vi "Boolean Array to Hex Values.vi"(11 "Array in":bool[][](array[boolean])) -> (3 "Array out":u8[](array[numeric]))   [LabVIEW 2026, in "LED Matrix.lvlib" / "Content.lvclass"]
uses:
  Content.lvclass
  Content.lvclass/Content.ctl
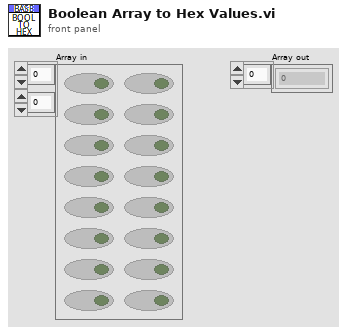
[diagram p1: front panel]
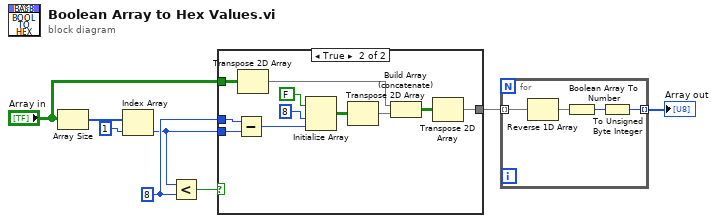
[diagram p0: block diagram]
diagram:
  w4 = 8 ("y")
  n1 = Array Size(array="Array in") -> (size(s)=w7:i32[])
  n2 = Index Array(array=w7, index=1) -> (element=w3:i32)
  n3 = Less?(x=w3, y=w4) -> (x < y?=w5:bool)
  n4 = case shown="True" w5 {
    tunnel: w4 -> [_ w20]
    tunnel: w3 -> [_ w19]
    tunnel: "Array in" -> [w9 w15]
    tunnel: [w9 w10] -> w1
    frame False {
    }
    frame True {
      n5 = Subtract(x=w20, y=w19) -> (x-y=w17:i32)
      n6 = Transpose 2D Array(2D array=w15) -> (transposed array=w12:bool[][])
      n7 = Initialize Array(FALSE, 8 ("dimension size"), w17) -> (w14:bool[][])
      n8 = Transpose 2D Array(2D array=w14) -> (transposed array=w13:bool[][])
      n9 = Build Array (concatenate)(w12, w13) -> (w11:bool[][])
      n10 = Transpose 2D Array(2D array=w11) -> (transposed array=w10:bool[][])
    }
  }
  n11 = for {
    tunnel: [w23] -> w8 mode=indexing
    tunnel: w1 -> [w21] mode=indexing
    n12 = Reverse 1D Array(array=w21) -> (reversed array=w22:bool[])
    n13 = Boolean Array To Number(Boolean array=w22) -> (number=w24:u32)
    n14 = To Unsigned Byte Integer(number=w24) -> (unsigned 8bit integer=w23:u8)
  }
  "Array out" <- w8
